vi "Fetch FFT Measurement Power.vi"(8 "error in (no error)":errorcluster, 9 "Result Type (Current)":i32(ring) items=["Current", "Average", "Maximum", "Minimum"], 10 "Instance (1)":i32=1, 11 "VISA resource name":refnum<visa-resource-name>) -> (0 "error out":errorcluster, 1 "Power":dbl[](array[numeric]) format="%^.3e", 2 "Reliability":i32, 3 "VISA resource name out":refnum<visa-resource-name>)   [LabVIEW 2020, in "Rohde&Schwarz CMXP GPRF.lvlib"]
doc: "Returns the \"FFT Spectrum Analyzer\" traces across the selected frequency span.\n\nAttributes:\nRSCMXPGPRF_ATTR_FETCH_FFT_MEASUREMENT_POWER_CURRENT\nRSCMXPGPRF_ATTR_FETCH_FFT_MEASUREMENT_POWER_AVERAGE\nRSCMXPGPRF_ATTR_FETCH_FFT_MEASUREMENT_POWER_MINIMUM\nRSCMXPGPRF_ATTR_FETCH_FFT_MEASUREMENT_POWER_MAXIMUM\n\nRemote-control commands:\nFETCh:GPRF:MEAS<i>:FFTSanalyzer:POWer:CURRent?\nFETCh:GPRF:MEAS<i>:FFTSanalyzer:POWer:AVERage?\nFETCh:GPRF:MEAS<i>:FFTSanalyzer:POWer:MINimum?\nFETCh:GPRF:MEAS<i>:FFTSanalyzer:POWer:MAXimum?"
uses:
  <instrlib>/Rohde&Schwarz CMXP GPRF/Rohde&Schwarz CMXP GPRF.lvlib
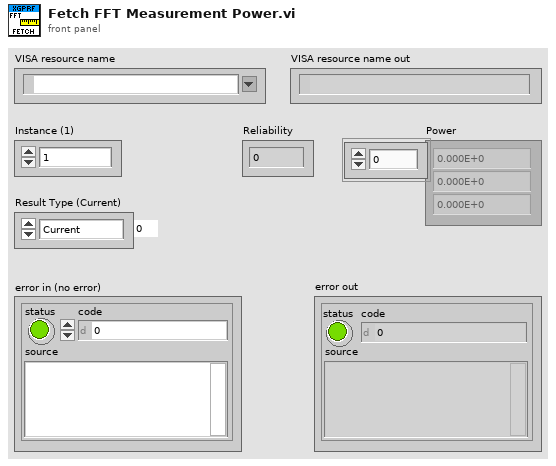
[diagram p1: front panel]
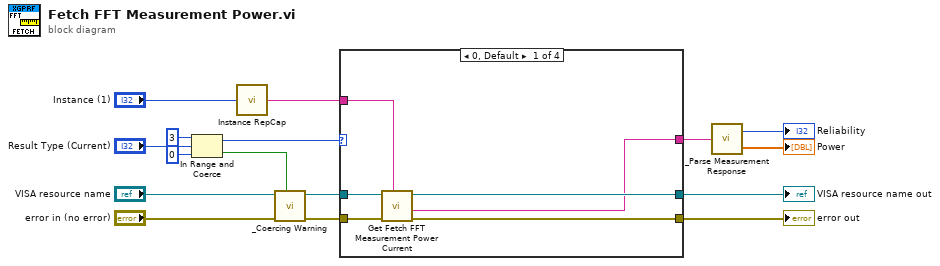
[diagram p0: block diagram]
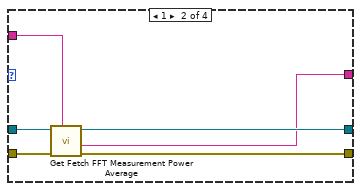
[diagram p2: hidden frame]
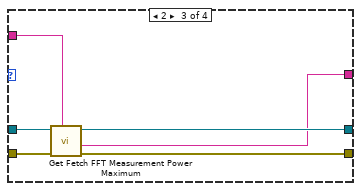
[diagram p3: hidden frame]
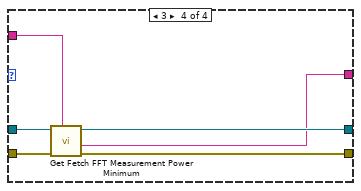
[diagram p4: hidden frame]
diagram:
  n1 = In Range and Coerce(upper limit=3, x="Result Type (Current)", lower limit=0) -> (coerced(x)=w14:i32, In Range?=w5:bool)
  n2 = call <instrlib>:"Instance RepCap.vi"("Instance in"="Instance (1)") -> ("Instance out"=w13:string)
  n3 = call <instrlib>:"_Coercing Warning.vi"("In Range?"=w5, "error in (no error)"="error in (no error)", "VISA resource name"="VISA resource name") -> ("error out"=w12:errorcluster, "VISA resource name out"=w11:refnum<visa-resource-name>)  [unwired: 7 in]
  n4 = case shown="0, Default" w14 {
    tunnel: w13 -> [w18 w24 w30 w36]
    tunnel: w12 -> [w22 w28 w34 w40]
    tunnel: w11 -> [w21 w27 w33 w39]
    tunnel: [w20 w26 w32 w38] -> w7
    tunnel: [w19 w25 w31 w37] -> w6
    tunnel: [w17 w23 w29 w35] -> w1
    frame 0, Default {
      n5 = call "Get Fetch FFT Measurement Power Current"("Repeated Capabilities"=w18, "error in (no error)"=w22, "instrument handle"=w21) -> ("error out"=w20:errorcluster, "Fetch FFT Measurement Power Current"=w17:string, "instrument handle out"=w19:refnum<visa-resource-name>)  [unwired: 6 in]
    }
    frame 1 {
      n6 = call "Get Fetch FFT Measurement Power Average"("Repeated Capabilities"=w24, "error in (no error)"=w28, "instrument handle"=w27) -> ("error out"=w26:errorcluster, "Fetch FFT Measurement Power Average"=w23:string, "instrument handle out"=w25:refnum<visa-resource-name>)  [unwired: 6 in]
    }
    frame 2 {
      n7 = call "Get Fetch FFT Measurement Power Maximum"("Repeated Capabilities"=w30, "error in (no error)"=w34, "instrument handle"=w33) -> ("error out"=w32:errorcluster, "Fetch FFT Measurement Power Maximum"=w29:string, "instrument handle out"=w31:refnum<visa-resource-name>)  [unwired: 6 in]
    }
    frame 3 {
      n8 = call "Get Fetch FFT Measurement Power Minimum"("Repeated Capabilities"=w36, "error in (no error)"=w40, "instrument handle"=w39) -> ("error out"=w38:errorcluster, "Fetch FFT Measurement Power Minimum"=w35:string, "instrument handle out"=w37:refnum<visa-resource-name>)  [unwired: 6 in]
    }
  }
  "error out" <- w7
  "VISA resource name out" <- w6
  n9 = call <instrlib>:"_Parse Measurement Response.vi"("String In"=w1) -> ("Reliability"=→"Reliability":i32, "Data"=→"Power":dbl[])
